vi "Test C.vi"(7 "Socket":i32, 8 "error in (no error)":errorcluster) -> (0 "error out":errorcluster)   [LabVIEW 2019, in "Multisocket Example(Station2).lvlib"]
uses:
  Multisocket Example(Station2).lvlib
  b65cedc0-6f88-47fe-863c-f92be18f8f6a.vi
  941f3686-130e-45b0-8e30-bc4649ace6bb.vi
  LVUT Global 1.vi
  <vilib>/Utility/Data Type/Get Type Information.vi
  <vilib>/Utility/error.llb/Trim Whitespace.vi
  Equal Value.vi
  Unit Test Engine Tools.lvlib
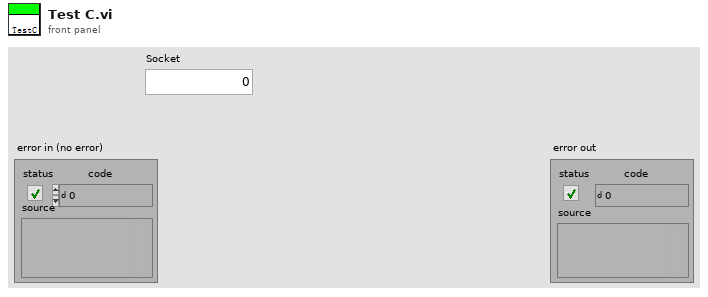
[diagram p1: front panel]
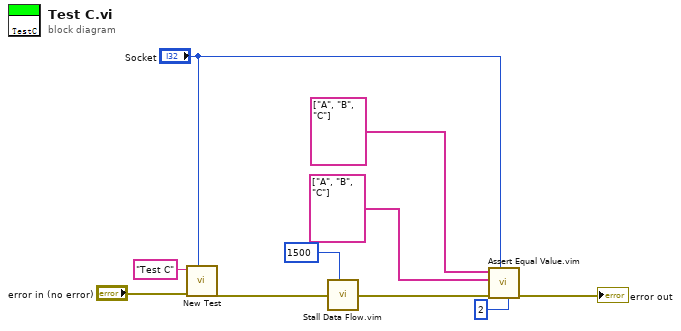
[diagram p0: block diagram]
diagram:
  n1 = call "New Test.vi"("Socket"="Socket", "error in (no error)"="error in (no error)", "Test"="Test C") -> ("error out"=w8:errorcluster)  [unwired: 8 in]
  n2 = call "Stall Data Flow.vim"("value in"=w8, "milliseconds to wait"=u32 1500) -> ("value out"=w5:errorcluster)  [unwired: 1 out]
  n3 = call "Assert Equal Value.vim"("precision (2)"=i16 2 ("precision (6)"), "Socket"="Socket", "error in (no error)"=w5, "Y"=string[] ["A", "B", "C"], "X"=string[] ["A", "B", "C"]) -> ("error out"=→"error out":errorcluster)  [unwired: 6 in]
